vi "error_log.vi"(1 "errors":u16[](array[numeric]), 2 "N modules":i32) -> ()   [LabVIEW 2021]
panel:
  in  "file basename":string="battery_error_"
  in  "path":path=path "C:/ni-rt/startup/datalog/error"
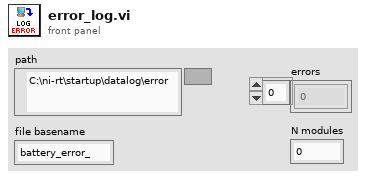
[diagram p1: front panel]
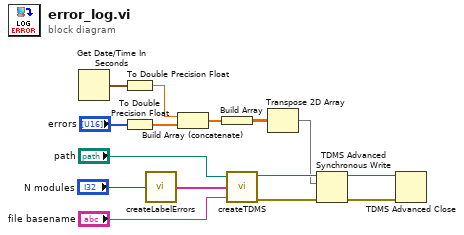
[diagram p0: block diagram]
diagram:
  n1 = Get Date/Time In Seconds() -> (seconds since 1Jan1904=w5:timestamp)
  n2 = To Double Precision Float(number=w5) -> (double precision float=w4:dbl)
  n3 = To Double Precision Float(number="errors") -> (double precision float=w3:dbl[])
  n4 = call "createLabelErrors.vi"("N modules"="N modules") -> ("labels (out)"=w11:string[])
  n5 = Build Array (concatenate)(w4, w3) -> (w2:dbl[])
  n6 = Build Array(w2) -> (w1:dbl[][])
  n7 = call "createTDMS.vi"("path"="path", "channel name(s)"=w11, "file basename"="file basename") -> ("Ref"=w10:refnum<k34>, "error out"=w9:errorcluster)  [unwired: 1 in, 1 out]
  n8 = Transpose 2D Array(2D array=w1) -> (transposed array=w8:dbl[][])
  n9 = TDMS Advanced Synchronous Write(8:w9, 10:w8, 11:w10) -> (0:w6:errorcluster, 3:w7:refnum<k34>)
  n10 = TDMS Advanced Close(8:w6, 11:w7) -> ()  [unwired: 2 in, 2 out]
